vi "Word_doc.vi"(8 "error in (no error)":errorcluster, 9 "report file path out":path=path "C:/Users/Joseph/Desktop/New folder/5.docx", 10 "Report in 2":path=path "C:/Users/Joseph/Desktop/RRATP000001 ATP_NAMER_60A_BDLC_60A _Vers 10_160816.doc", 11 "Report in 1":path=path "C:/KineticksTester/N30_00000_200817_1048.docx") -> (0 "error out":errorcluster)   [LabVIEW 2017]
uses:
  <vilib>/Utility/NIReport.llb/NI_report.lvclass
  <vilib>/Utility/NIReport.llb/Word/NI_Word.lvclass
  <vilib>/addons/_office/NI_ReportGenerationToolkit.lvlib
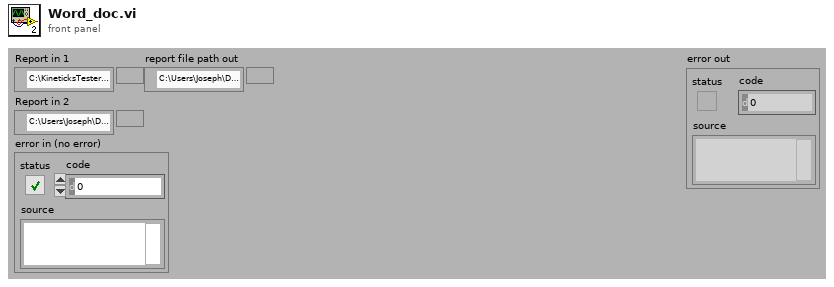
[diagram p1: front panel]
types:
  T1 = enum16{"Standard Report", "HTML", "Word", "Excel"}
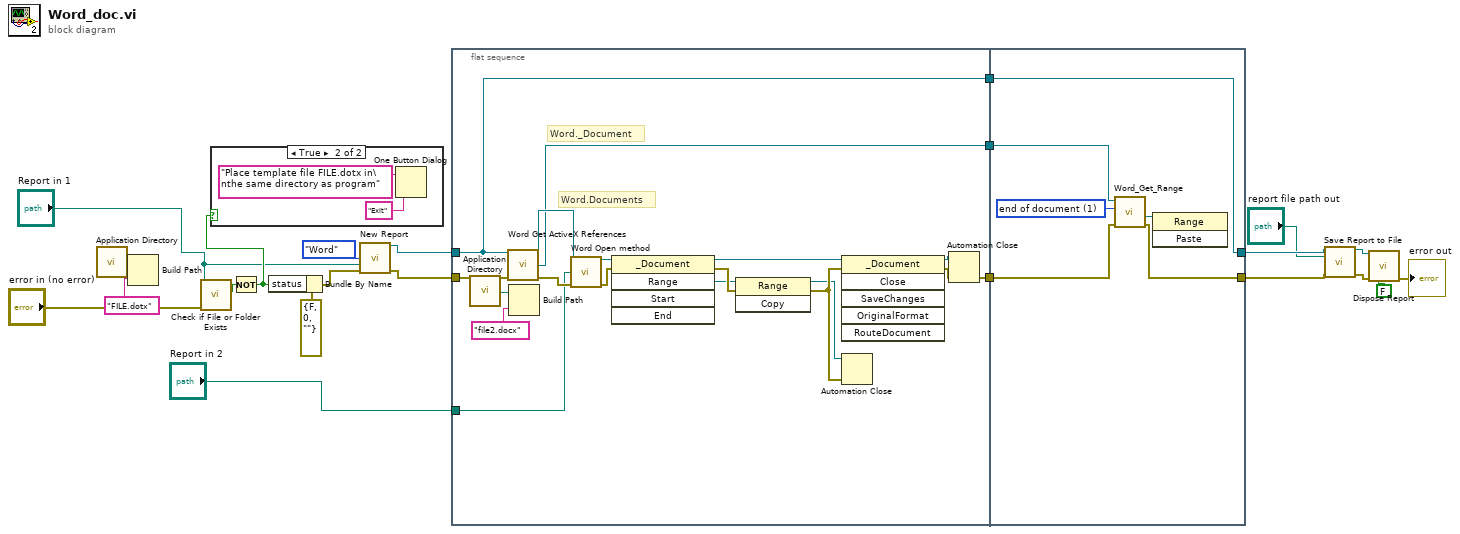
[diagram p0: block diagram]
diagram:
  n1 = call <vilib>:"Application Directory.vi"() -> ("Application Directory"=w13:path)
  n2 = Build Path(base path=w13, name or relative path="FILE.dotx" ("text")) -> ()  [unwired: 1 out]
  n3 = call <vilib>:"Check if File or Folder Exists.vi"("error in (no error)"="error in (no error)", "path"="Report in 1") -> ("file or folder exists?"=w18:bool)  [unwired: 7 in, 2 out]
  n4 = Not(x=w18) -> (.not. x?=w14:bool)
  n5 = case shown="True" w14 {
    frame False {
    }
    frame True {
      n6 = One Button Dialog(message="Place template file FILE.dotx in\nthe same directory as program", button name ("OK")="Exit") -> ()  [unwired: 1 out]
    }
  }
  n7 = Bundle By Name(cluster=errorcluster {"status"=FALSE, "code"=0, "source"=""} ("error in (no error)"), "status"=w14) -> (w19:errorcluster)
  n8 = call <vilib>:"New Report.vi"("report type"=T1."Word", "template (empty)"="Report in 1", "error in (no error)"=w19) -> ("report out"=w17:refnum<class "NI_report.lvclass">, "error out"=w16:errorcluster)  [unwired: 11 in]
  n9 = flat-sequence {
    tunnel: w17 -> [w26]
    tunnel: w16 -> [w42]
    tunnel: [w27] -> w12
    tunnel: [w28] -> w11
    tunnel: [w26] -> w10
    tunnel: "Report in 2" -> [w25]
    tunnel: w12 -> [w46]
    tunnel: [w44] -> w7
    tunnel: [w43] -> w6
    tunnel: w11 -> [w45]
    tunnel: w10 -> [w44]
    frame #0 {
      # "Word.Documents"
      # "Word._Document"
      n10 = call <vilib>:"Application Directory.vi"() -> ("Application Directory"=w29:path)
      n11 = call <vilib>:"Word Get ActiveX References.vi"("report in"=w26, "error in (no error)"=w42) -> ("Word.Documents"=w33:refnum<k7>, "Word._Document"=w28:refnum<k7>, "error out"=w38:errorcluster)  [unwired: 7 in, 4 out]
      n12 = Build Path(base path=w29, name or relative path="file2.docx" ("text")) -> ()  [unwired: 1 out]
      n13 = call <vilib>:"Word Open method.vi"("Word.Documents"=w33, "FileName"=w25, "error in (no error)"=w38) -> ("Open"=w34:refnum<k7>, "error out"=w39:errorcluster)  [unwired: 11 out]
      n14 = invoke on="Range" class="_Document" method="Range"(reference=w34, error in=w39) -> (reference out=w35:refnum<k7>, error out=w37:errorcluster, "Range"=w32:refnum<k7>)  [unwired: 3 in, 2 out]
      n15 = invoke on="Copy" class="Range" method="Copy"(reference=w32, error in=w37) -> (reference out=w31:refnum<k7>, error out=w41:errorcluster)  [unwired: 1 in, 1 out]
      n16 = invoke on="Close" class="_Document" method="Close"(reference=w35, error in=w41) -> (reference out=w36:refnum<k7>, error out=w40:errorcluster)  [unwired: 4 in, 4 out]
      n17 = Automation Close(3:w41, 5:w31) -> ()  [unwired: 1 out]
      n18 = Automation Close(3:w40, 5:w36) -> (0:w27:errorcluster)
    }
    frame #1 {
      w48 = u16 1 items=["begining of document", "end of document", "bookmark", "Custom"] ("insertion point")
      n19 = call <vilib>:"Word_Get_Range.vi"("error in"=w46, "insertion point"=w48, "document in"=w45) -> ("error out (no error)"=w43:errorcluster, "range"=w47:refnum<k7>)  [unwired: 3 in, 4 out]
      n20 = invoke class="Range" method="Paste"(reference=w47) -> ()  [unwired: 2 in, 3 out]
    }
  }
  n21 = call-dynamic "Save Report to File.vi"("report in"=w7, "report file path"="report file path out", "error in (no error)"=w6) -> ("report out"=w4:refnum<class "NI_report.lvclass">, "error out"=w5:errorcluster)  [unwired: 11 in]
  n22 = call-dynamic "Dispose Report.vi"("report in"=w4, "error in (no error)"=w5, "close report? (T)"=FALSE) -> ("error out"=→"error out":errorcluster)  [unwired: 12 in]
